vi "Main.vi"(11 "Module Admin":refnum<class "Delacor_lib_QMH_Module Admin.lvclass">) -> ()   [LabVIEW 2026, in "Front Panel Emulator.lvlib"]
doc: "This template is based off of the Queued Message Handler design pattern and the Queued Message Handler project template that ships with LabVIEW.\n\nThe main difference is that the queue is private to this module and communication between modules is performed via Broadcast and Request events.\n\nRequest events are wrapped in public API methods and are handled in the Event Handling Loop (EHL) of this VI. Any module can register for Broadcast events sent by this module. The EHL generates messages based on user interface actions.\n\nThe Message Handling Loop (MHL) processes messages generated by the EHL, or by other messages. The messages are string values, so new messages can be added easily to the Message Cases case structure in the MHL. Each message cluster can also provide an optional value for Message Data, which is a variant that can be converted to whatever message-specific data is required.\n_____\nBased on DQMH Dev Tools: Project Template 7.1.2.1547."
uses:
  Front Panel Emulator.lvlib
  <vilib>/Delacor/Delacor QMH/Libraries/Module Admin_class/Delacor_lib_QMH_Module Admin.lvclass
  Module Data--cluster.ctl
  Stop Argument--cluster.ctl
  <vilib>/Delacor/Delacor QMH/Libraries/Message Queue_class/Delacor_lib_QMH_Message Queue.lvclass/Delacor_lib_QMH_Message Queue.ctl
  <vilib>/Delacor/Delacor QMH/Libraries/Module Admin_class/Delacor_lib_QMH_Module Admin.lvclass/Delacor_lib_QMH_Module Admin.ctl
  Update Temperature Argument--cluster.ctl
  Update Humidity Argument--cluster.ctl
  <vilib>/Utility/miscctls.llb/LVPointTypeDef.ctl
  <vilib>/Delacor/Delacor QMH/Libraries/Message Queue_class/Delacor_lib_QMH_Enqueue Message (Single).vi
  <vilib>/Delacor/Delacor QMH/Libraries/Module Admin_class/Delacor_lib_QMH_Get External Launch.vi
  <vilib>/Delacor/Delacor QMH/Libraries/Message Queue_class/Delacor_lib_QMH_Message Queue.lvclass
panel:
  in  "Position":dbl(knob) min=0.0 max=180.0 scale=0.0..180.0
  out "LCD":string
  out "error out":errorcluster
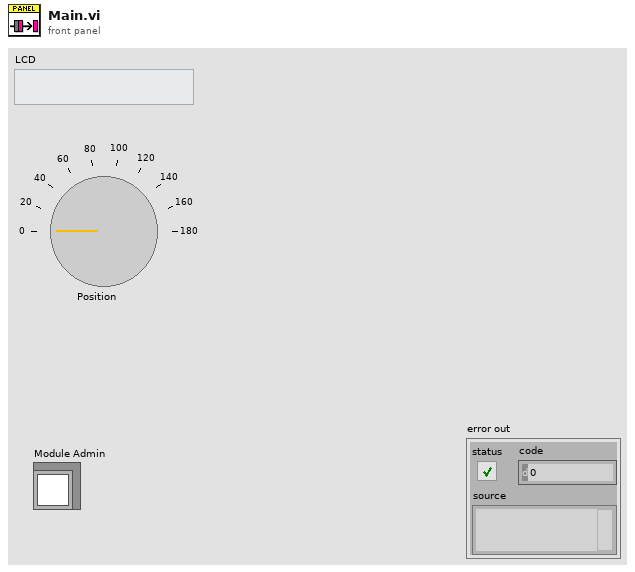
[diagram p1: front panel]
types:
  T1 = typedef "Front Panel Emulator.lvlib/Request Events--cluster.ctl" = cluster{"Stop Module":refnum<user-event>, "Show Panel":refnum<user-event>, "Hide Panel":refnum<user-event>, "Get Module Execution Status":refnum<user-event>, "Show Diagram":refnum<user-event>, "Update Temperature":refnum<user-event>, "Update Humidity":refnum<user-event>}
  T2 = typedef "Front Panel Emulator.lvlib/Module Data--cluster.ctl" = cluster{"Status":string, "Temperature":dbl, "RH":dbl, "Position":dbl}
  T3 = enum32{"invalid lock state", "Not Locked", "Locked (No Password)", "Password-protected"}
  T4 = typedef "Front Panel Emulator.lvlib/Stop Argument--cluster.ctl" = cluster{"Origin":string, "Exit via Stop Module Req?":bool, "Wait for Module to stop?":bool}
  T5 = typedef "Front Panel Emulator.lvlib/Update Temperature Argument--cluster.ctl" = cluster{"Temperature":dbl}
  T6 = typedef "Front Panel Emulator.lvlib/Update Humidity Argument--cluster.ctl" = cluster{"Relative Humidity":dbl}
  T7 = typedef "LVPointTypeDef.ctl" = cluster{"Horizontal":i16, "Vertical":i16}
  T8 = enum32{"Invalid", "Standard", "Closed", "Hidden", "Minimized", "Maximized"}
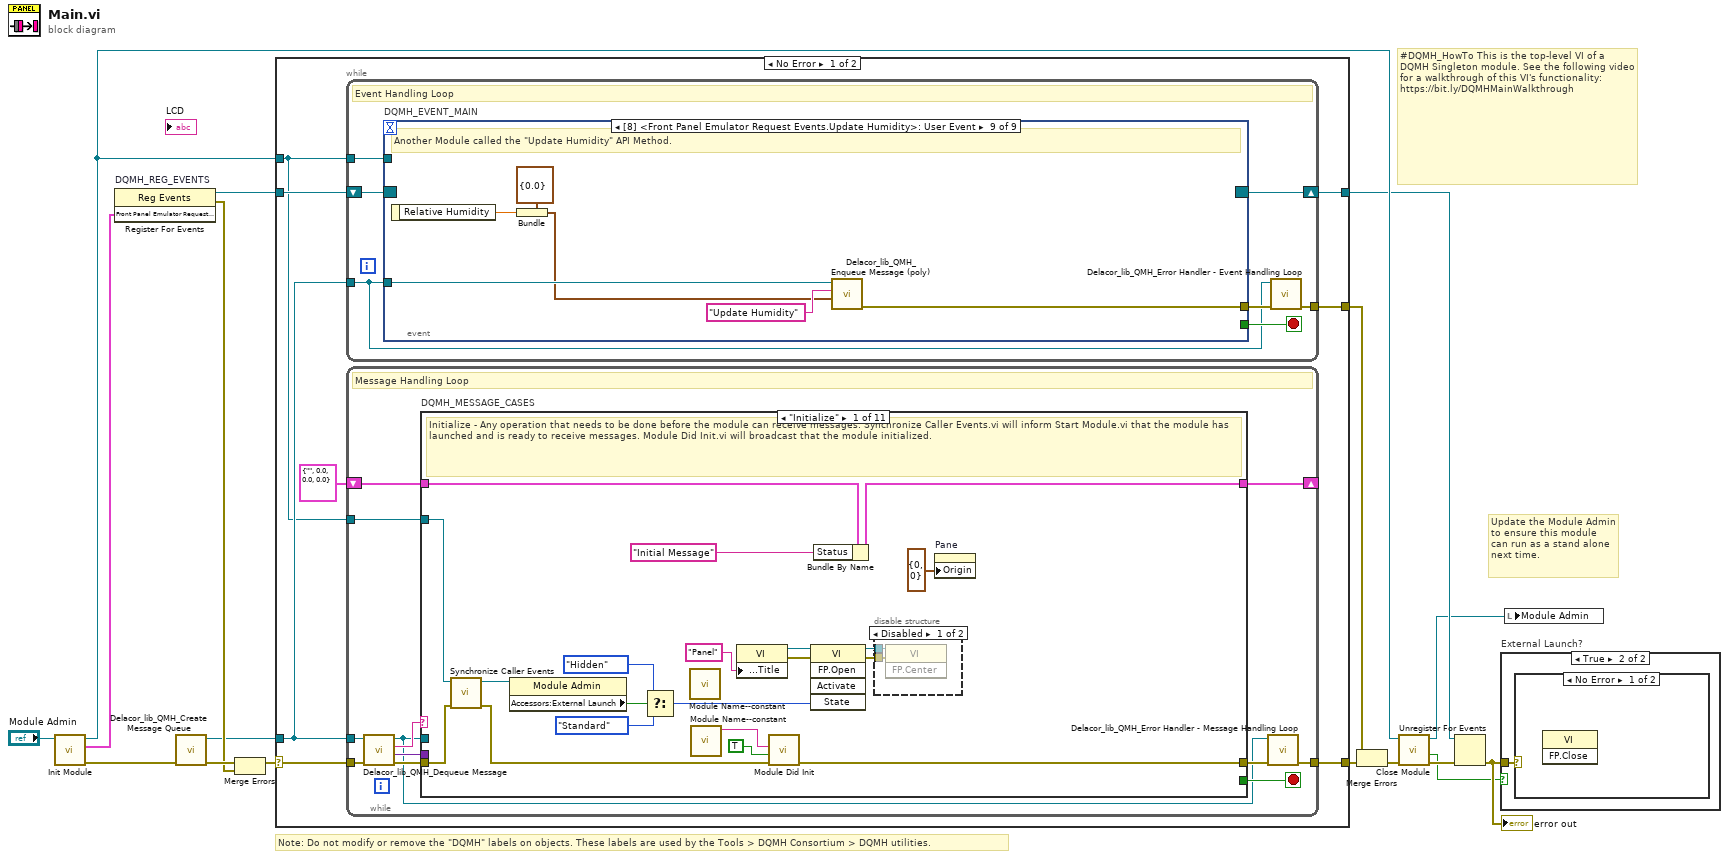
[diagram p0: block diagram]
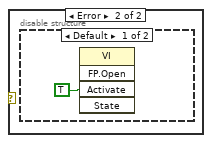
[diagram p3: hidden frame]
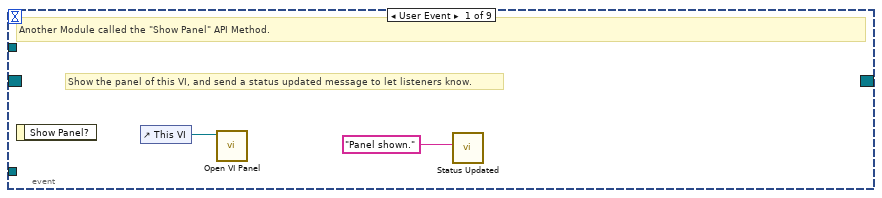
[diagram p5: hidden frame]
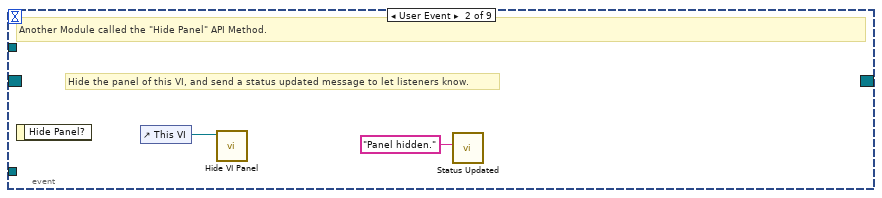
[diagram p6: hidden frame]
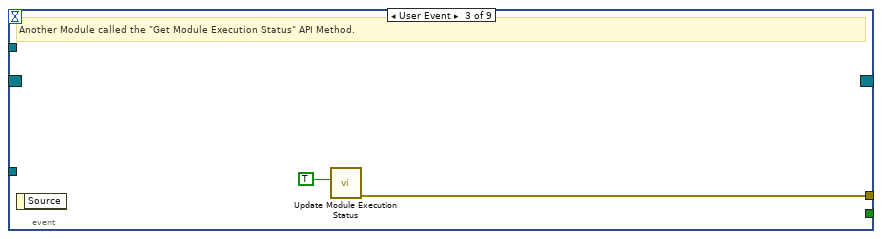
[diagram p7: hidden frame]
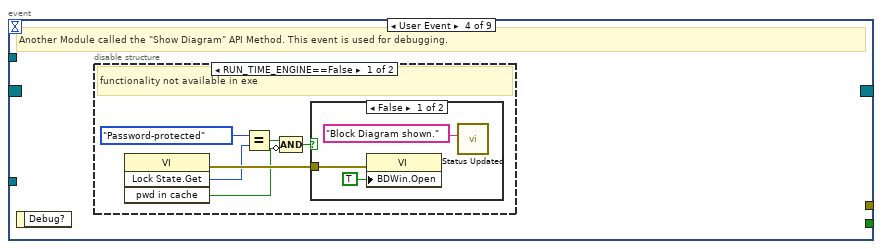
[diagram p8: hidden frame]
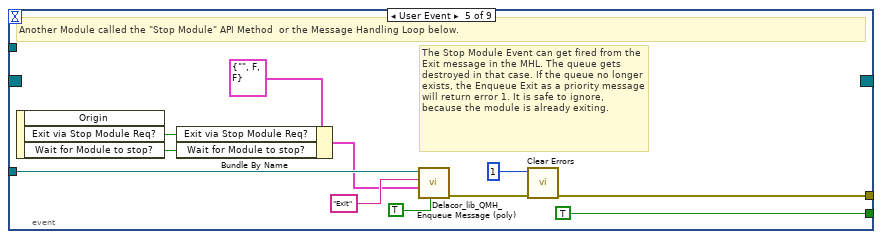
[diagram p11: hidden frame]
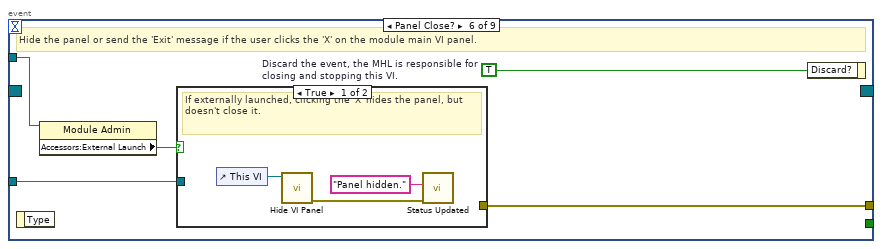
[diagram p12: hidden frame]
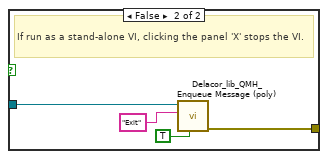
[diagram p13: hidden frame]
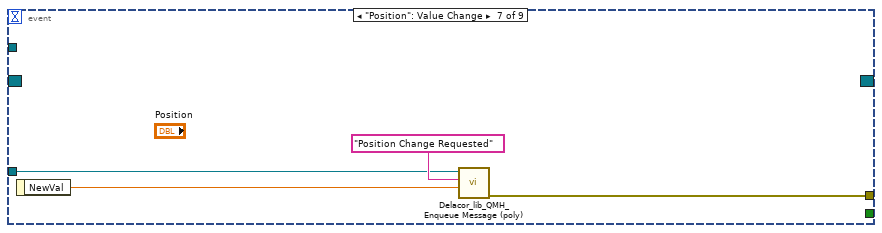
[diagram p14: hidden frame]
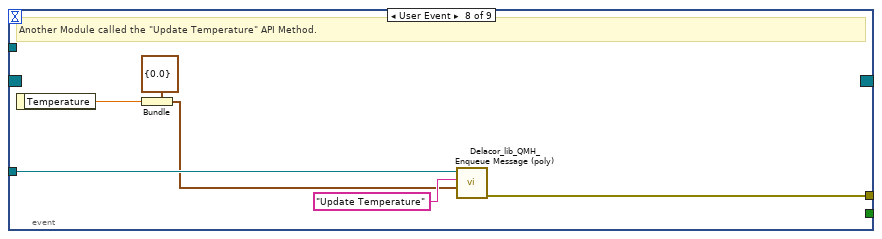
[diagram p15: hidden frame]
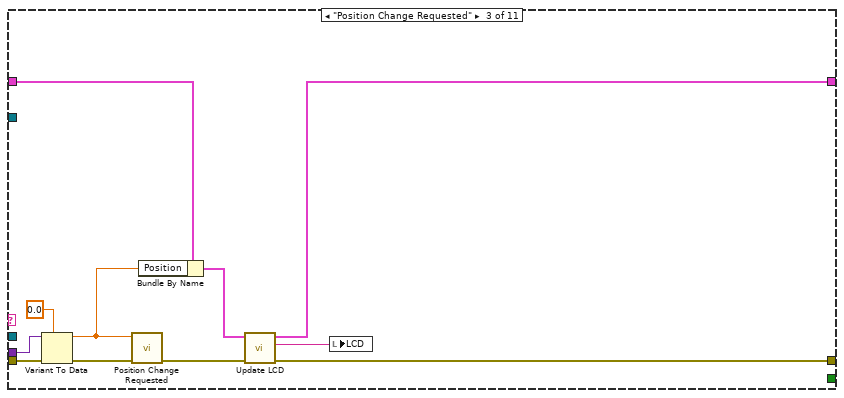
[diagram p18: hidden frame]
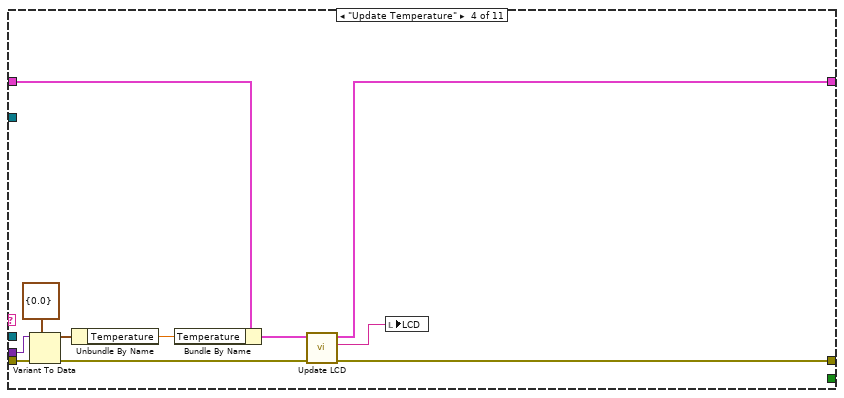
[diagram p19: hidden frame]
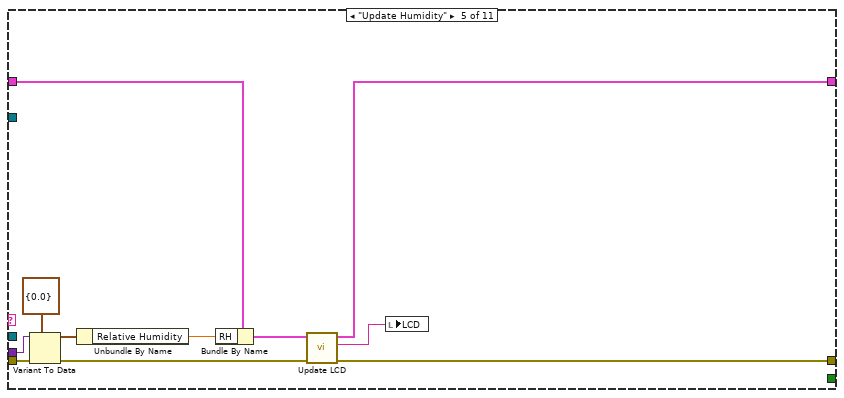
[diagram p20: hidden frame]
diagram:
  # "#DQMH_HowTo This is the top-level VI of a DQMH Singleton module. See the following video for a walkthrough of this VI's functionality: https://bit.ly/DQMHMainWalkthrough"
  # "Note: Do not modify or remove the \"DQMH\" labels on objects. These labels are used by the Tools > DQMH Consortium > DQMH utilities."
  # "Update the Module Admin to ensure this module can run as a stand alone next time."
  n1 = call "Init Module.vi"("Singleton Module Admin in"="Module Admin") -> ("error out"=w16:errorcluster, "Front Panel Emulator Request Events"=w5:T1, "Singleton Module Admin out"=w8:refnum<class "Delacor_lib_QMH_Module Admin.lvclass">)  [unwired: 8 in]
  n2 = register-events "DQMH_REG_EVENTS"(w5) -> (reference out=w6:refnum<event-registration>, error out=w9:errorcluster)  [unwired: 2 in]
  n3 = call <vilib>:"Delacor_lib_QMH_Create Message Queue.vi"("error in"=w16) -> ("error out"=w11:errorcluster, "Message Queue"=w4:refnum<class "Delacor_lib_QMH_Message Queue.lvclass">)  [unwired: 9 in]
  n4 = Merge Errors(w11, w9) -> (w10:errorcluster)
  n5 = case shown="No Error" w10 {
    selector: w10 -> [w23 w219]
    tunnel: [w25 w218] -> w17
    tunnel: [w22 w217] -> w7
    tunnel: w6 -> [w20 w217]
    tunnel: w4 -> [w19 w212]
    tunnel: [w24 _] -> w14
    tunnel: w8 -> [w18 w213]
    frame No Error {
      n6 = while {
        tunnel: w19 -> [w26]
        shift-right: [w29] -> w22
        shift-left: w20 -> [w30]
        tunnel: [w31] -> w24
        tunnel: w18 -> [w27]
        stop <- w28 stop-if-true
        # "Event Handling Loop"
        n7 = event "DQMH_EVENT_MAIN" shown="[8] <Front Panel Emulator Request Events.Update Humidity>: User Event" {
          selector: w30 -> [_ _ _ _ _ _ _ _ _]
          dyn-events: [_ _ _ _ _ _ _ _ _] -> w29
          timeout: _ -> [_ _ _ _ _ _ _ _ _]
          tunnel: [_ _ _ _ TRUE ("Discard?") _ _ _ _] -> w28
          tunnel: w26 -> [_ _ _ _ w54 w61 w73 w80 w86]
          tunnel: [_ _ w38 _ w57 w63 w72 w75 w81] -> w32
          tunnel: w27 -> [_ _ _ _ _ w60 _ _ _]
          event User Event {
            # "Show the panel of this VI, and send a status updated message to let listeners know."
            # "Another Module called the \"Show Panel\" API Method."
            n8 = event-data() -> ()  [unwired: 1 in, 1 out]
            n9 = control-ref of="This VI"() -> (w34:refnum<vi>)
            n10 = call "Open VI Panel.vi"("VI"=w34) -> ()  [unwired: 10 in, 1 out]
            n11 = call "Status Updated.vi"("Status"="Panel shown." ("format string")) -> ()  [unwired: 10 in, 1 out]
          }
          event User Event {
            # "Hide the panel of this VI, and send a status updated message to let listeners know."
            # "Another Module called the \"Hide Panel\" API Method."
            n12 = event-data() -> ()  [unwired: 1 in, 1 out]
            n13 = control-ref of="This VI"() -> (w36:refnum<vi>)
            n14 = call "Hide VI Panel.vi"("VI"=w36) -> ()  [unwired: 10 in, 1 out]
            n15 = call "Status Updated.vi"("Status"="Panel hidden." ("format string")) -> ()  [unwired: 10 in, 1 out]
          }
          event User Event {
            # "Another Module called the \"Get Module Execution Status\" API Method."
            n16 = event-data() -> ()  [unwired: 1 in, 1 out]
            n17 = call "Update Module Execution Status.vi"("Running?"=TRUE) -> ("error out"=w38:errorcluster)  [unwired: 10 in]
          }
          event User Event {
            # "Another Module called the \"Show Diagram\" API Method. This event is used for debugging."
            n18 = event-data() -> ()  [unwired: 1 in, 1 out]
            n19 = disable-structure shown="RUN_TIME_ENGINE==False" {
              frame condition #0 (active) {
                # "functionality not available in exe"
                n20 = invoke on="Invoke Node" class="VI" method="Lock State.Get"() -> (error out=w44:errorcluster, "Get Lock State"=w43:T3, "pwd in cache"=w40:bool)  [unwired: 4 in, 1 out]
                n21 = Equal?(x=T3."Password-protected", y=w43) -> (x = y?=w41:bool)
                n22 = Compound Arithmetic op=AND(w41, invert w40) -> (w39:bool)
                n23 = case shown="False" w39 {
                  tunnel: w44 -> [w47 _]
                  frame False {
                    n24 = property on="Property Node" class="VI"(error in=w47, "BDWin.Open"=TRUE ("Block Diagram Window:Open")) -> ()  [unwired: 1 in, 2 out]
                    n25 = call "Status Updated.vi"("Status"="Block Diagram shown." ("format string")) -> ()  [unwired: 10 in, 1 out]
                  }
                  frame True {
                    # "Password-protected VI, and the password is not in the cache. Do not show the diagram."
                  }
                }
              }
              frame condition #1 {
              }
            }
          }
          event User Event {
            # "The Stop Module Event can get fired from the Exit message in the MHL. The queue gets destroyed in that case. If the queue no longer exists, the Enqueue Exit as a priority message will return error 1. It is safe to ignore, because the module is already exiting."
            # "Another Module called the \"Stop Module\" API Method  or the Message Handling Loop below."
            n26 = event-data() -> ("Exit via Stop Module Req?"=w50:bool, "Wait for Module to stop?"=w49:bool)  [unwired: 1 in, 1 out]
            n27 = Bundle By Name(cluster=T4 {"Origin"="", "Exit via Stop Module Req?"=FALSE, "Wait for Module to stop?"=FALSE} ("Stop Argument"), "Exit via Stop Module Req?"=w50, "Wait for Module to stop?"=w49) -> (w48:T4)
            n28 = call-poly <vilib>:"Delacor_lib_QMH_Enqueue Message (poly).vi"("Priority Message? (F)"=TRUE, "Message Data"=w48, "Message"="Exit", "Message Queue in"=w54) -> ("error out"=w58:errorcluster)  [unwired: 6 in, 1 out]
            n29 = call <vilib>:"Clear Errors.vi"("error in (no error)"=w58, "specific error code to clear (0: all)"=1) -> ("error out"=w57:errorcluster)  [unwired: 4 in, 1 out]
          }
          event Panel Close? {
            w62 = TRUE  # Discard the event, the MHL is responsible for closing and stopping this VI.
            # "Hide the panel or send the 'Exit' message if the user clicks the 'X' on the module main VI panel."
            n30 = event-data() -> ()  [unwired: 1 in, 1 out]
            n31 = property on="Property Node" class="Module Admin"(reference=w60) -> ("Accessors:External Launch"=w59:bool)  [unwired: 1 in, 2 out]
            n32 = case shown="True" w59 {
              tunnel: w61 -> [_ w69]
              tunnel: [_ w70] -> w63
              frame True {
                # "If externally launched, clicking the 'X' hides the panel, but doesn't close it."
                n33 = control-ref of="This VI"() -> (w66:refnum<vi>)
                n34 = call "Hide VI Panel.vi"("VI"=w66) -> ("error out"=w64:errorcluster)  [unwired: 10 in]
                n35 = call "Status Updated.vi"("error in"=w64, "Status"="Panel hidden." ("format string")) -> ()  [unwired: 9 in, 1 out]
              }
              frame False {
                # "If run as a stand-alone VI, clicking the panel 'X' stops the VI."
                n36 = call-poly <vilib>:"Delacor_lib_QMH_Enqueue Message (poly).vi"("Priority Message? (F)"=TRUE, "Message"="Exit", "Message Queue in"=w69) -> ("error out"=w70:errorcluster)  [unwired: 7 in, 1 out]
              }
            }
            n37 = event-data ("Event Filter Node")("Discard?"=w62) -> ()  [unwired: 1 in, 1 out]
          }
          event "Position": Value Change {
            n38 = event-data() -> ("NewVal"=w71:dbl)  [unwired: 1 in]
            n39 = call-poly <vilib>:"Delacor_lib_QMH_Enqueue Message (poly).vi"("Message Data"=w71, "Message"="Position Change Requested", "Message Queue in"=w73) -> ("error out"=w72:errorcluster)  [unwired: 7 in, 1 out]
          }
          event User Event {
            # "Another Module called the \"Update Temperature\" API Method."
            n40 = event-data() -> ("Temperature"=w76:dbl)  [unwired: 1 in]
            n41 = Bundle(cluster=T5 {"Temperature"=0.0} ("Update Temperature Argument"), "Temperature"=w76) -> (w77:T5)
            n42 = call-poly <vilib>:"Delacor_lib_QMH_Enqueue Message (poly).vi"("Message Data"=w77, "Message"="Update Temperature", "Message Queue in"=w80) -> ("error out"=w75:errorcluster)  [unwired: 7 in, 1 out]
          }
          event User Event {
            # "Another Module called the \"Update Humidity\" API Method."
            n43 = event-data() -> ("Relative Humidity"=w82:dbl)  [unwired: 1 in]
            n44 = Bundle(cluster=T6 {"Relative Humidity"=0.0} ("Update Humidity Argument"), "Relative Humidity"=w82) -> (w83:T6)
            n45 = call-poly <vilib>:"Delacor_lib_QMH_Enqueue Message (poly).vi"("Message Data"=w83, "Message"="Update Humidity", "Message Queue in"=w86) -> ("error out"=w81:errorcluster)  [unwired: 7 in, 1 out]
          }
        }
        n46 = call-dynamic "Delacor_lib_QMH_Error Handler - Event Handling Loop.vi"("error in"=w32, "Message Queue in"=w26) -> ("dup error in"=w31:errorcluster)  [unwired: 8 in, 1 out]
      }
      n47 = while {
        tunnel: w19 -> [w87]
        shift-right: [w95] -> _
        shift-left: T2 {"Status"="", "Temperature"=0.0, "RH"=0.0, "Position"=0.0} ("Data Cluster") -> [w96]
        tunnel: w23 -> [w98]
        tunnel: [w90] -> w25
        tunnel: w18 -> [w91]
        stop <- w94 stop-if-true
        # "Message Handling Loop"
        n48 = call-dynamic "Delacor_lib_QMH_Dequeue Message.vi"("error in"=w98, "Message Queue in"=w87) -> ("error out"=w97:errorcluster, "Message Data"=w92:variant, "Message"=w93:string, "Message Queue out"=w88:refnum<class "Delacor_lib_QMH_Message Queue.lvclass">)  [unwired: 6 in]
        n49 = case "DQMH_MESSAGE_CASES" shown="\"Initialize\"" w93 {
          selector: w93 -> [_ _ _ _ _ _ _ _ _ _ w207]
          tunnel: w88 -> [_ _ _ _ _ _ _ _ w173 w195 _]
          tunnel: w97 -> [w116 w122 w128 w144 w155 w158 w160 w169 w180 w201 w210]
          tunnel: [w114 w122 w124 w134 w145 w157 w160 w168 w176 w196 w211] -> w89
          tunnel: w96 -> [w106 w121 w133 w136 w147 w156 w159 w166 w175 w194 w208]
          tunnel: [w105 w121 w125 w137 w148 w156 w159 w166 w175 w194 w208] -> w95
          tunnel: [_ _ _ _ _ _ _ _ _ w193 _] -> w94
          tunnel: w92 -> [_ _ w132 w143 w154 _ _ _ w174 w192 _]
          tunnel: w91 -> [w107 _ _ _ _ _ _ _ w172 w187 _]
          frame "Initialize" {
            # "Initialize - Any operation that needs to be done before the module can receive messages. Synchronize Caller Events.vi will inform Start Module.vi that the module has launched and is ready to receive messages. Module Did Init.vi will broadcast that the module initialized."
            n50 = call "Synchronize Caller Events.vi"("error in"=w116, "Singleton Module Admin in"=w107) -> ("error out"=w115:errorcluster, "Singleton Module Admin out"=w102:refnum<class "Delacor_lib_QMH_Module Admin.lvclass">)  [unwired: 8 in]
            n51 = property on="Property Node" class="Module Admin"(reference=w102) -> ("Accessors:External Launch"=w111:bool)  [unwired: 1 in, 2 out]
            n52 = Select(t=T8."Hidden" ("State"), s=w111, f=T8."Standard" ("State")) -> (s? t:f=w108:T8)
            n53 = call "Module Name--constant.vi"() -> ()  [unwired: 11 in, 1 out]
            n54 = call "Module Name--constant.vi"() -> ("Module Name"=w103:string)  [unwired: 11 in]
            n55 = property on="Property Node" class="VI"("Front Panel.Title"="Panel" ("Front Panel Window:Title")) -> (reference out=w113:refnum<vi>, error out=w118:errorcluster)  [unwired: 2 in]
            n56 = call "Module Did Init.vi"("error in"=w115, "Initialized?"=TRUE, "Origin"=w103) -> ("error out"=w114:errorcluster)  [unwired: 8 in]
            n57 = invoke on="Invoke Node" class="VI" method="FP.Open"(reference=w113, error in=w118, "State"=w108) -> (reference out=w112:refnum<vi>, error out=w117:errorcluster)  [unwired: 2 in, 3 out]
            n58 = Bundle By Name(cluster=w106, "Status"="Initial Message" ("Initial Message")) -> (w105:T2)
            n59 = disable-structure shown="Disabled" {
              disable-tunnel: w117 -> [w120 _]
              disable-tunnel: w112 -> [w119 _]
              frame Disabled {
                n60 = invoke on="Invoke Node" class="VI" method="FP.Center"(reference=w119, error in=w120) -> ()  [unwired: 1 in, 3 out]
              }
              frame Enabled {
              }
            }
            n61 = property on="Pane" class="Pane"("Origin"=T7 {"Horizontal"=0, "Vertical"=0}) -> ()  [unwired: 2 in, 2 out]
          }
          frame "---Module Specific---" {
            # "Separator -- The following cases handle messages specific to this Module."
          }
          frame "Position Change Requested" {
            n62 = Variant To Data(error in=w128, type=0.0 ("NewVal"), Variant=w132) -> (data=w126:dbl, error out=w129:errorcluster)
            n63 = call "Position Change Requested.vi"("error in"=w129, "Position"=w126) -> ("error out"=w130:errorcluster)  [unwired: 9 in]
            n64 = Bundle By Name(cluster=w133, "Position"=w126) -> (w127:T2)
            n65 = call "Update LCD.vi"("error in"=w130, "Data Cluster"=w127) -> ("error out"=w124:errorcluster, "LCD"=w123:string, "Module Data"=w125:T2)  [unwired: 7 in]
            n66 = local write "LCD"(w123) -> ()
          }
          frame "Update Temperature" {
            n67 = Variant To Data(error in=w144, type=T5 {"Temperature"=0.0} ("Update Temperature Argument"), Variant=w143) -> (data=w141:T5, error out=w135:errorcluster)
            n68 = Unbundle By Name(w141) -> ("Temperature"=w138:dbl)
            n69 = Bundle By Name(cluster=w136, "Temperature"=w138) -> (w140:T2)
            n70 = call "Update LCD.vi"("error in"=w135, "Data Cluster"=w140) -> ("error out"=w134:errorcluster, "LCD"=w139:string, "Module Data"=w137:T2)  [unwired: 7 in]
            n71 = local write "LCD"(w139) -> ()
          }
          frame "Update Humidity" {
            n72 = Variant To Data(error in=w155, type=T6 {"Relative Humidity"=0.0} ("Update Humidity Argument"), Variant=w154) -> (data=w152:T6, error out=w146:errorcluster)
            n73 = Unbundle By Name(w152) -> ("Relative Humidity"=w149:dbl)
            n74 = Bundle By Name(cluster=w147, "RH"=w149) -> (w151:T2)
            n75 = call "Update LCD.vi"("error in"=w146, "Data Cluster"=w151) -> ("error out"=w145:errorcluster, "LCD"=w150:string, "Module Data"=w148:T2)  [unwired: 7 in]
            n76 = local write "LCD"(w150) -> ()
          }
          frame "---Copy This Frame---" {
            # "Duplicate this frame when creating new messages.  Change this comment in the duplicated frame to describe this message."
            n77 = Merge Errors(w158) -> (w157:errorcluster)
          }
          frame "---Exit and Error Handling---" {
            # "Separator - The following cases handle errors and exit messages."
          }
          frame "Simulate MHL Error" {
            # "#DQMH_HowTo The 'Simulate MHL Error' button  illustrates how the MHL handles errors. This event is instructional in nature and can be removed."
            # "Simulate an error occurring at the MHL"
            n78 = call "Module Name--constant.vi"() -> ("Module Name"=w162:string)  [unwired: 11 in]
            n79 = Format Into String(format string="Simulated error originating at Message Handling Loop in %s", w162) -> (resulting string=w163:string)  [unwired: 2 in, 1 out]
            n80 = call <vilib>:"Error Cluster From Error Code.vi"("show call chain? (False)"=TRUE, "error message (\"\")"=w163, "error code (0)"=5001) -> ("error out"=w167:errorcluster)  [unwired: 6 in]
            n81 = Merge Errors(w169, w167) -> (w168:errorcluster)
          }
          frame "Error" {
            # "#DQMH_CodeRecommended - If the module is running in standalone mode (External Launch = FALSE), this code will pop up an error dialog and call the 'Exit' message if an error occurs. Add more fine-grained error management here."
            # "Error - Check the error message data and respond accordingly. This message is sent by the \"Error Handler\" VIs at the end of each loop in this application."
            n82 = property on="Property Node" class="Module Admin"(reference=w172) -> ("Accessors:External Launch"=w171:bool)  [unwired: 1 in, 2 out]
            n83 = Variant To Data(error in=w180, type=errorcluster {"status"=FALSE, "code"=0, "source"=""} ("error constant"), Variant=w174) -> (data=w170:errorcluster, error out=w178:errorcluster)
            n84 = local write "error out"(w170) -> ()
            n85 = call "Error Reported.vi"("Error"=w170) -> ()  [unwired: 10 in, 1 out]
            n86 = case shown="False" w171 {
              tunnel: [w185 _] -> w177
              tunnel: w173 -> [w183 _]
              tunnel: w170 -> [w184 _]
              frame False {
                n87 = disable-structure shown="Default" {
                  disable-tunnel: w184 -> [w186 _]
                  frame condition #0 (active) {
                    # "If the module is running standalone, then pop up an error dialog and call the \"Exit\" message."
                    n88 = call <vilib>:"Simple Error Handler.vi"("error in (no error)"=w186) -> ()  [unwired: 4 in, 5 out]
                  }
                  frame condition #1 {
                    # "To prevent the Simple Error Handler VI from being loaded (e.g. when deploying to a Real-Time target), add the Conditional Disable Symbol \"DQMH_Disable_SEH\" to your project and set it to TRUE."
                  }
                }
                n89 = call-poly <vilib>:"Delacor_lib_QMH_Enqueue Message (poly).vi"("Priority Message? (F)"=TRUE, "Message"="Exit", "Message Queue in"=w183) -> ("error out"=w185:errorcluster)  [unwired: 7 in, 1 out]
              }
              frame True {
                # "If the module was launched externally, calling the Error Reported broadcast VI is the only action performed by the \"Error\" message. The module's caller can then process the error appropriately."
              }
            }
            n90 = Merge Errors(w178, w177) -> (w176:errorcluster)
          }
          frame "Exit" {
            w191 = 91  # 91: not all Exit messages will have an argument
            w193 = TRUE  # Stop the VI
            # "Release the message queue reference"
            # "#DQMH_CodeNeeded - Add any required cleanup code here."
            # "Exit - Exit the application."
            n91 = Variant To Data(error in=w201, type=T4 {"Origin"="", "Exit via Stop Module Req?"=FALSE, "Wait for Module to stop?"=FALSE} ("Stop Argument"), Variant=w192) -> (data=w189:T4, error out=w198:errorcluster)
            n92 = call <vilib>:"Clear Errors.vi"("error in (no error)"=w198, "specific error code to clear (0: all)"=w191) -> ("error out"=w200:errorcluster)  [unwired: 4 in, 1 out]
            n93 = control-ref of="This VI"() -> (w188:refnum<vi>)
            n94 = call-dynamic "Delacor_lib_QMH_Release Message Queue.vi"("error in"=w200, "Message Queue"=w195) -> ("error out"=w199:errorcluster)  [unwired: 9 in]
            n95 = call "Handle Exit.vi"("Stop Argument"=w189, "Admin in"=w187, "VI reference"=w188) -> ("error out"=w197:errorcluster)  [unwired: 7 in, 1 out]
            n96 = Merge Errors(w199, w197) -> (w196:errorcluster)
            n97 = call "Error Reported.vi"("Error"=w196) -> ()  [unwired: 10 in, 1 out]
          }
          frame Default {
            # "'Default' case only runs if there is a message that isn't defined in any of the other cases.  Output a programming error."
            n98 = call "Module Name--constant.vi"() -> ("Module Name"=w206:string)  [unwired: 11 in]
            n99 = Format Into String(format string="The invalid message string \"%s\" was received in the Message Handling Loop for module \"%s\".", w207, w206) -> (resulting string=w202:string)  [unwired: 2 in, 1 out]
            n100 = call <vilib>:"Error Cluster From Error Code.vi"("show call chain? (False)"=TRUE, "error message (\"\")"=w202, "error code (0)"=1) -> ("error out"=w209:errorcluster)  [unwired: 6 in]
            n101 = Merge Errors(w210, w209) -> (w211:errorcluster)
          }
        }
        n102 = call-dynamic "Delacor_lib_QMH_Error Handler - Message Handling Loop.vi"("error in"=w89, "Message Queue in"=w88) -> ("dup error in"=w90:errorcluster)  [unwired: 8 in, 1 out]
      }
    }
    frame Error {
      # "Synchronize Caller Events.vi will inform Start Module.vi that the module has launched and will let the code calling Start Module.vi register for broadcasts and would permit the caller receive the broadcast that an error occurred at launch time."
      n103 = call-dynamic "Delacor_lib_QMH_Release Message Queue.vi"("error in"=w219, "Message Queue"=w212) -> ("error out"=w218:errorcluster)  [unwired: 9 in]
      n104 = call "Synchronize Caller Events.vi"("Singleton Module Admin in"=w213) -> ("error out"=w220:errorcluster)  [unwired: 9 in, 1 out]
      n105 = call "Module Name--constant.vi"() -> ("Module Name"=w216:string)  [unwired: 11 in]
      n106 = Format Into String(format string="An error occurred during initialization. %s is no longer running.", w216) -> (resulting string=w214:string)  [unwired: 2 in, 1 out]
      n107 = Merge Errors(w218, w220) -> (w221:errorcluster)
      n108 = call "Error Reported.vi"("Additional Information"=w214, "Error"=w221) -> ()  [unwired: 9 in, 1 out]
    }
  }
  n109 = Merge Errors(w14, w17) -> (w13:errorcluster)
  n110 = call "Close Module.vi"("error in"=w13, "Module Admin in"=w8) -> ("error out"=w15:errorcluster, "External Launch"=w1:bool, "Module Admin out"=w2:refnum<class "Delacor_lib_QMH_Module Admin.lvclass">)  [unwired: 7 in]
  n111 = Unregister For Events(event registration refnum=w7, error in=w15) -> (error out=w12:errorcluster)
  "error out" <- w12
  n112 = case "External Launch?" shown="True" w1 {
    tunnel: w12 -> [_ w222]
    frame False {
    }
    frame True {
      n113 = case shown="No Error" w222 {
        frame No Error {
          n114 = invoke on="Invoke Node" class="VI" method="FP.Close"() -> ()  [unwired: 3 in, 3 out]
        }
        frame Error {
          n115 = disable-structure shown="Default" {
            frame condition #0 (active) {
              n116 = invoke class="VI" method="FP.Open"("Activate"=TRUE ("Activate?")) -> ()  [unwired: 4 in, 5 out]
            }
            frame condition #1 {
              # "Don't show panel on error if running inside a built EXE."
            }
          }
        }
      }
    }
  }
  n117 = local write "Module Admin"(w2) -> ()
